vi "Autonomous Independent.vi"() -> ()   [LabVIEW 2015]
doc: "This VI is called when autonomous begins, and will automatically be terminated when autonomous ends. You can carry out timed or sensor driven robot movement independently without needing to return to the caller."
uses:
  Autonomous/Typedef/MainStates.ctl
  Autonomous/SubVI/Auton System Monitor.ctl
  Autonomous/Typedef/Defences.ctl
  Autonomous/Typedef/AutonRefType.ctl
  <vilib>/Rock Robotics/WPI/RobotDrive/WPI_RobotDriveDevRef.ctl
  <vilib>/Rock Robotics/WPI/MotorControl/WPI_MotorControlDeviceRef.ctl
  <vilib>/Rock Robotics/WPI/MotorControl/WPI_MotorControlType.ctl
  <vilib>/Rock Robotics/SystemInterfaces/DIO/FPGA_DIOPWMChannel.ctl
  <vilib>/Rock Robotics/WPI/PWM/WPI_PWMDeadband.ctl
  <vilib>/Rock Robotics/WPI/CAN/Jaguar/SubVIs/WPI_CANJaguar_ControlMode.ctl
  <vilib>/Rock Robotics/WPI/CAN/TalonSRX/WPI_CANTalonSRX_APIControlMode.ctl
  <vilib>/Rock Robotics/WPI/Encoder/WPI_EncoderDevRef.ctl
  <vilib>/Rock Robotics/SystemInterfaces/Encoder/FPGA_EncoderIdx.ctl
  <vilib>/Rock Robotics/SystemInterfaces/Counter/FPGA_CounterCtrSystemIndex.ctl
  <vilib>/Rock Robotics/WPI/Encoder/WPI_EncoderType.ctl
  <vilib>/Rock Robotics/WPI/Switch/WPI_SwitchDevRef.ctl
  <vilib>/Rock Robotics/SystemInterfaces/DIO/FPGA_DIOChannel.ctl
  NavX/TypeDefs/Z900_navX_DeviceTypeDef.ctl
  NavX/TypeDefs/Z900_navX_ProtocolTypeDef.ctl
  NavX/TypeDefs/Z900_navX_NotifyPacketTypeDef.ctl
  NavX/TypeDefs/Z900_navX_ActionTypeDef.ctl
  <vilib>/Rock Robotics/WPI/Potentiometer/WPI_PotentiometerDevRef.ctl
  <vilib>/Rock Robotics/SystemInterfaces/AI/FPGA_AIChannel.ctl
  <vilib>/Rock Robotics/Network Tables/NT Read String.vi
  <vilib>/Rock Robotics/WPI/Utilities/WPI_GetSetVariantRefNum.vi
  <vilib>/Rock Robotics/Network Tables/NT Write String.vi
  Robot Global Data.vi
  <vilib>/Rock Robotics/WPI/RobotDrive/WPI_RobotDriveArcadeDrive_Standard(NoSaturation).vi
  NavX/navX Library v2.lvlib
  <vilib>/ptbypt/NI_PtbyPt.lvlib
  ArmController/ArmController.lvlib
panel:
  in  "Channels":i32[](array[numeric]) caption="Drive Channels to Monitor"
  out "System Monitor Config":T1={"Brownout?"=FALSE, "Current Max?"=FALSE, "System Max Current"=240.0, "Min Voltage"=6.2, "Drive Motor Max Current"=40.0, "Drive Motor Time (s)"=3.5}
  out "System Monitor":T2(graph)
  in  "RUN":bool=TRUE
  in  "stop":bool
  in  "Test Case":T3
  in  "Test Case":bool
  in  "Auton Steps":T4(tab)
  in  "Gyro Turn Output Range":cluster{"output high":dbl, "output low":dbl}={"output high"=0.8, "output low"=-0.8}
  in  "Gyro PID gains":T5={"proportional gain (Kc)"=0.0005, "integral time (Ti, min)"=0.0, "derivative time (Td, min)"=0.0} {"derivative time (Td, min)" format="%.3f"; "integral time (Ti, min)" format="%.3f"; "proportional gain (Kc)" format="%.5f"}
  in  "Target Position":dbl=158.0 format="%#_13g"
  in  "Speed":dbl=0.75
  out "Encoder Difference":dbl=9.15275203438432
  out "Angle Error":dbl=0.004439899999999999
  in  "output rate (EGU/min)":dbl=1.0 format="%.2f"
  in  "Hit Wall Distance":dbl=60.0 format="%#_13g"
  in  "Hit wall speed":dbl=0.35
  in  "Gyro Turn Output Range 2":cluster{"output high":dbl, "output low":dbl}={"output high"=0.5, "output low"=-0.5}
  in  "Backup Distance":dbl=-24.0 format="%#_13g"
  in  "Hit wall speed 2":dbl=0.45
  in  "Gyro Turn Output Range 3":cluster{"output high":dbl, "output low":dbl}={"output high"=0.65, "output low"=-0.65}
  in  "Max Vel (in/s)":dbl=50.0
  in  "Kp_Yaw 2":dbl=0.0005 format="%#_13g"
  in  "Max Accel (in/s^2)":dbl=400.0
  in  "output range 3":cluster{"output high":dbl, "output low":dbl}={"output high"=0.7, "output low"=-0.7}
  in  "Kv 3":dbl=0.012
  in  "Period (s) 3":dbl=0.005
  in  "Ka 3":dbl
  in  "PID gains 3":T5
  out "Waveform Chart":T2(graph)
  in  "Kv":dbl=0.012
  in  "Ka":dbl
  in  "Period (s)":dbl=0.005
  in  "output range":cluster{"output high":dbl, "output low":dbl}={"output high"=1.0, "output low"=-1.0} {"output low" format="%.2f"; "output high" format="%.2f"}
  in  "PID gains":T5 {"derivative time (Td, min)" format="%.3f"; "integral time (Ti, min)" format="%.3f"; "proportional gain (Kc)" format="%.3f"}
  in  "Target Position 2":dbl=60.0 format="%#_13g"
  in  "Max Acceleration":dbl=400.0
  in  "Max Velocity":dbl=75.0
  in  "Kp_Yaw":dbl
  in  "Scrub Factor":dbl=0.6
  out "Waveform Chart 2":T2(graph)
  in  "Max Velocity 2":dbl=60.0
  in  "Max Acceleration 2":dbl=600.0
  in  "Target Angle (deg)":dbl=-180.0 format="%#_13g"
  in  "output range 2":cluster{"output high":dbl, "output low":dbl}={"output high"=1.0, "output low"=-1.0} {"output low" format="%.2f"; "output high" format="%.2f"}
  in  "Period (s) 2":dbl=0.005
  in  "PID gains 2":T5={"proportional gain (Kc)"=0.005, "integral time (Ti, min)"=0.0, "derivative time (Td, min)"=0.0} {"derivative time (Td, min)" format="%.3f"; "integral time (Ti, min)" format="%.3f"; "proportional gain (Kc)" format="%.3f"}
  in  "Ka 2":dbl=0.0045
  in  "Kv 2":dbl=0.012
  out "CDF":T6(graph)
  in  "CDF Pos":dbl=0.608 format="%#_13g"
  in  "Speed 1":dbl=-0.34 format="%#_13g"
  in  "CDF Detect":dbl=0.585 format="%#_13g"
  in  "Start Wait":u32=1500
  in  "Drive Time x 20ms":i32=300
  in  "Drive Val":dbl format="%#_13g"
  # "Just above motor brownout"
  # "Hit Driversation Wall"
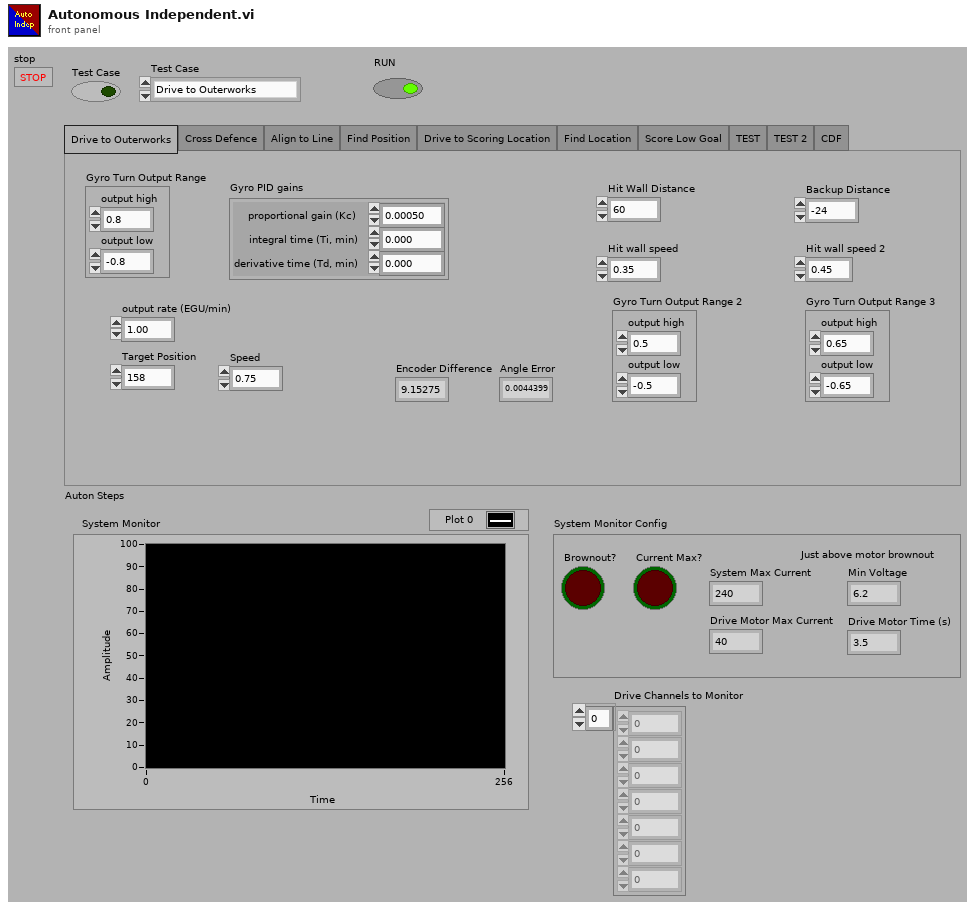
[diagram p1: front panel]
types:
  T1 = typedef "Auton System Monitor.ctl" = cluster{"Brownout?":bool, "Current Max?":bool, "System Max Current":dbl, "Min Voltage":dbl, "Drive Motor Max Current":dbl, "Drive Motor Time (s)":dbl}
  T2 = cluster{"Distance":dbl, "dx/dt":dbl, "dx/dt":dbl, "dx/dt":dbl}
  T3 = typedef "MainStates.ctl" = enum16{"Drive to Outerworks", "Cross Defence", "Align to Line", "Turn to Goal", "Find Position", "Find Distance", "Drive to Scoring Location", "Score Low Goal", "SquareToField", "Hit Driver Station Wall", "Drive Back to Position", "CDF", "Cleanup", "_TEST_Profile", "_TEST_TurnProfile", "_TEST_Impulse", "Error"}
  T4 = enum32{"Drive to Outerworks", "Cross Defence", "Align to Line", "Find Position", "Drive to Scoring Location", "Find Location", "Score Low Goal", "TEST", "TEST 2", "CDF"}
  T5 = cluster{"proportional gain (Kc)":dbl, "integral time (Ti, min)":dbl, "derivative time (Td, min)":dbl}
  T6 = cluster{"Normalized Value":dbl, "CDF Detect":dbl}
  T7 = typedef "AutonRefType.ctl" = cluster{"Starting Pos":u32, "Defence":T8, "Drivetrain":T9, "State":T3, "Encoder Right":T17, "Encoder Left":T17, "Line Sensor":T21, "navX":T23, "Front Arm":T25, "Start Time":u32, "State Vars":variant}
  T8 = typedef "Defences.ctl" = enum16{"Low Bar", "Chivel De Fris", "Sally Port", "Portcullis", "Draw Bridge", "Moat", "Rough Terrain", "Ramparts", "Rock Wall"}
  T9 = typedef "WPI_RobotDriveDevRef.ctl" = cluster{"DevStatus":errorcluster, "Motors[]":T10[], "Square Inputs":bool, "Max Output":dbl}
  T10 = typedef "WPI_MotorControlDeviceRef.ctl" = cluster{"DeviceStatus":errorcluster, "Type":T11, "PWM":cluster{"PWM Channel":T12, "DeadBand":T13}, "CAN":cluster{"Device Number":u8, "Control Mode":T14, "Semaphore":T15, "Max Vout":dbl, "TalonSRX Control Mode":T16}, "Invert":bool}
  T11 = typedef "WPI_MotorControlType.ctl" = enum16{"PWM", "CAN", "CANTalonSRX"}
  T12 = typedef "FPGA_DIOPWMChannel.ctl" = enum8{"PWM 0", "PWM 1", "PWM 2", "PWM 3", "PWM 4", "PWM 5", "PWM 6", "PWM 7", "PWM 8", "PWM 9", "PWM MXP 0", "PWM MXP 1", "PWM MXP 2", "PWM MXP 3", "PWM MXP 4", "PWM MXP 5", "PWM MXP 6", "PWM MXP 7", "PWM MXP 8", "PWM MXP 9", "Invalid"}
  T13 = typedef "WPI_PWMDeadband.ctl" = cluster{"Name":string, "maxPositivePwm":i32, "minPositivePwm":i32, "centerPwm":i32, "maxNegativePwm":i32, "minNegativePwm":i32, "angularRange":u16}
  T14 = typedef "WPI_CANJaguar_ControlMode.ctl" = enum8{"Percent VBus", "Current", "Speed", "Position", "Voltage"}
  T15 = typedef "Semaphore RefNum" = refnum<k1>
  T16 = typedef "WPI_CANTalonSRX_APIControlMode.ctl" = enum8{"Percent VBus", "Speed", "Position", "Slave", "Unchanged / Invalid", "Voltage Compensation", "Current", "Motion Profile"}
  T17 = typedef "WPI_EncoderDevRef.ctl" = cluster{"DevStatus":errorcluster, "EncoderIndex":T18, "CounterIndex":T19, "DistancePerCount":dbl, "Decoding Type":T20}
  T18 = typedef "FPGA_EncoderIdx.ctl" = enum8{"Enc 0", "Enc 1", "Enc 2", "Enc 3", "Enc 4", "Enc 5", "Enc 6", "Enc 7", "Invalid"}
  T19 = typedef "FPGA_CounterCtrSystemIndex.ctl" = enum8{"Ctr 0", "Ctr 1", "Ctr 2", "Ctr 3", "Ctr 4", "Ctr 5", "Ctr 6", "Ctr 7", "Invalid"}
  T20 = typedef "WPI_EncoderType.ctl" = enum16{"1x", "2x", "4x"}
  T21 = typedef "WPI_SwitchDevRef.ctl" = cluster{"DevStatus":errorcluster, "DIO Channel":T22, "CntIndex":T19, "Normally Closed":bool}
  T22 = typedef "FPGA_DIOChannel.ctl" = enum8{"DIO 0", "DIO 1", "DIO 2", "DIO 3", "DIO 4", "DIO 5", "DIO 6", "DIO 7", "DIO 8", "DIO 9", "DIO MXP 0", "DIO MXP 1", "DIO MXP 2", "DIO MXP 3", "DIO MXP 4", "DIO MXP 5", "DIO MXP 6", "DIO MXP 7", "DIO MXP 8", "DIO MXP 9", "DIO MXP 10", "DIO MXP 11", "DIO MXP 12", "DIO MXP 13", "DIO MXP 14", "DIO MXP 15", "Invalid"}
  T23 = typedef "navX Library v2.lvlib/Z900_navX_DeviceTypeDef.ctl" = cluster{"Interface":cluster{"Protocol":T24, "Update Rate (4Hz-60Hz)":u8, "navX Open TypeDef":variant}, "Notify Packet":refnum<notifier>, "Loop VI Refnum":refnum<vi>, "Ready to Close Occurrence Refnum":refnum<k4>}
  T24 = typedef "navX Library v2.lvlib/Z900_navX_ProtocolTypeDef.ctl" = enum16{"SERIAL", "I2C", "SPI"}
  T25 = typedef "WPI_PotentiometerDevRef.ctl" = cluster{"DevStatus":errorcluster, "Analog Channel":T26, "Invert Output":bool}
  T26 = typedef "FPGA_AIChannel.ctl" = enum8{"AI 0", "AI 1", "AI 2", "AI 3", "AI MXP 0", "AI MXP 1", "AI MXP 2", "AI MXP 3", "Invalid"}
  T27 = typedef "Motion Profile.ctl" = cluster{"Position":dbl[], "Velocity":dbl[], "Time":dbl[], "Acceleration":dbl[]}
  T28 = cluster{"Yaw":dbl, "Roll":dbl, "Pitch":dbl, "Heading":dbl, "Fused Heading":dbl}
  T29 = cluster{"Down":dbl, "Pickup":dbl, "Shoot":dbl, "Turtle":dbl, "Intake Transfer":dbl, "Hang":dbl}
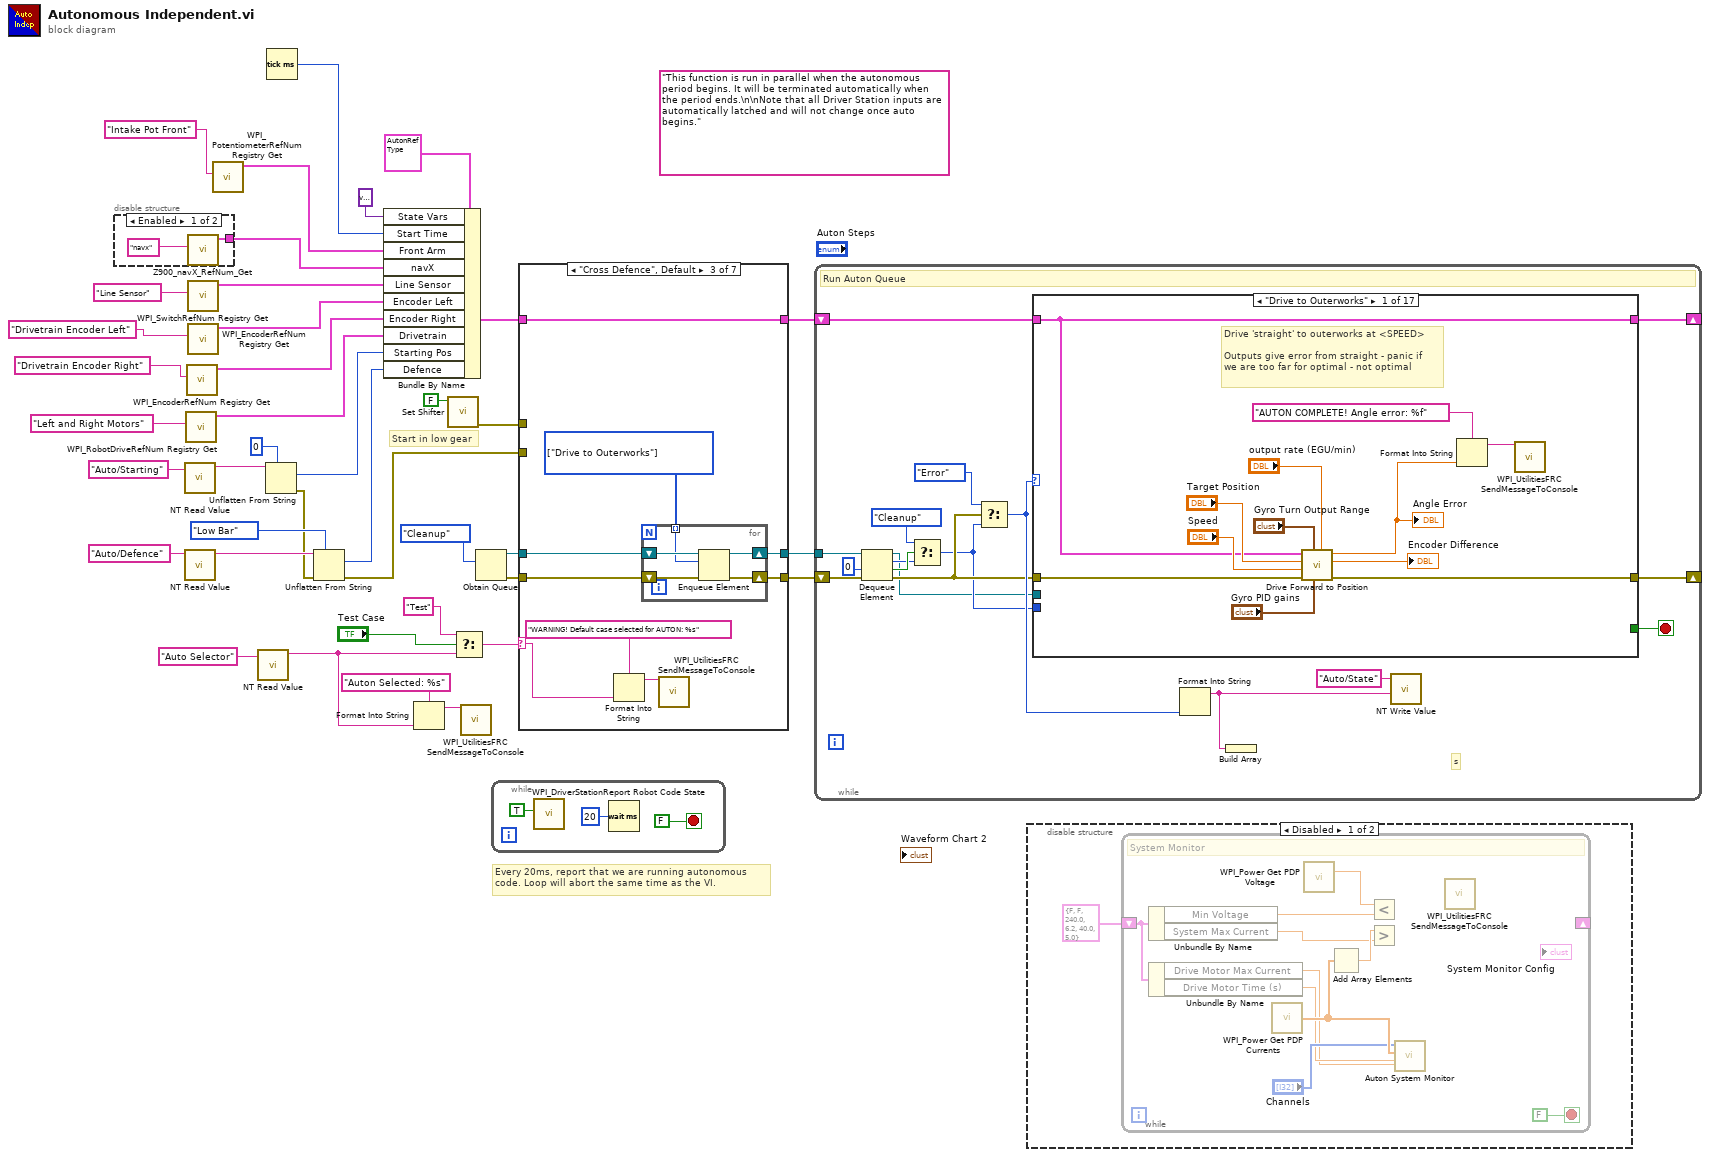
[diagram p0: block diagram]
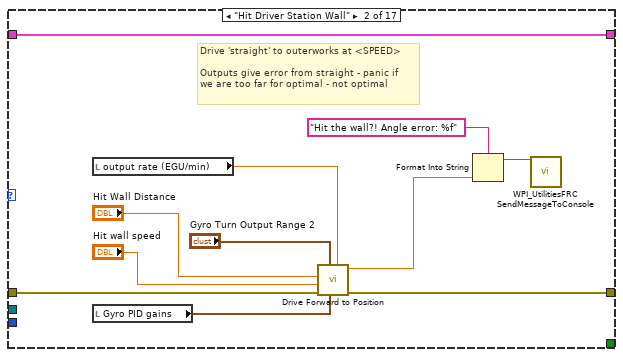
[diagram p4: hidden frame]
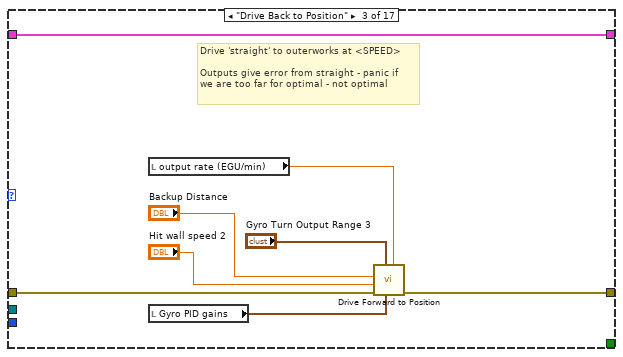
[diagram p5: hidden frame]
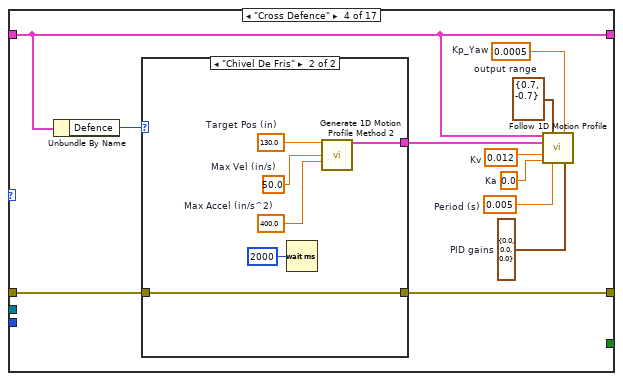
[diagram p6: hidden frame]
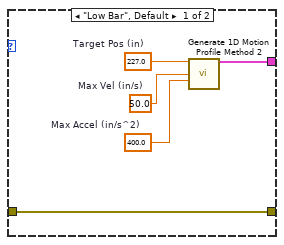
[diagram p7: hidden frame]
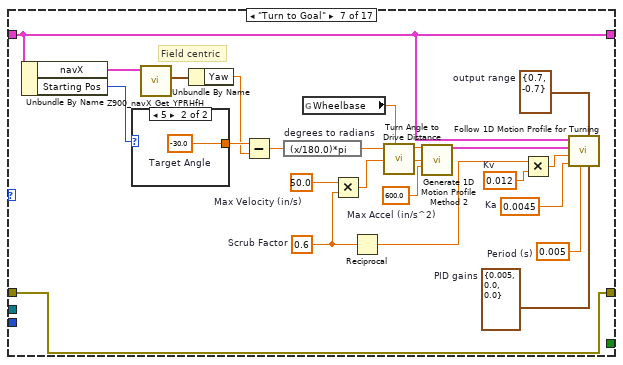
[diagram p10: hidden frame]
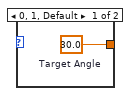
[diagram p11: hidden frame]
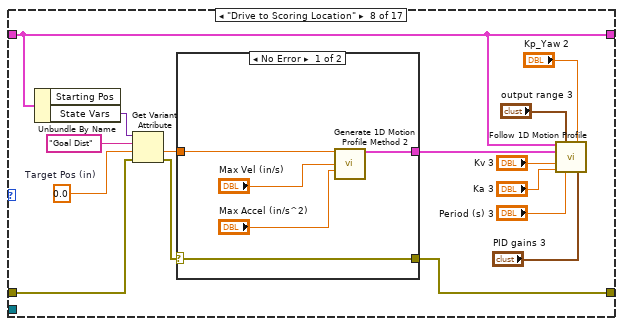
[diagram p12: hidden frame]
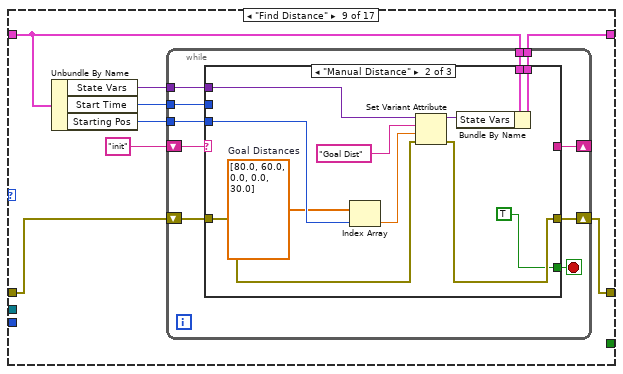
[diagram p14: hidden frame]
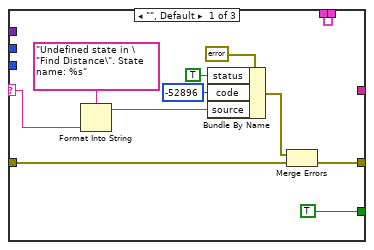
[diagram p15: hidden frame]
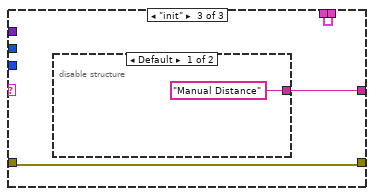
[diagram p16: hidden frame]
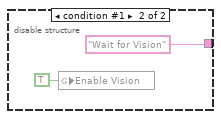
[diagram p17: hidden frame]
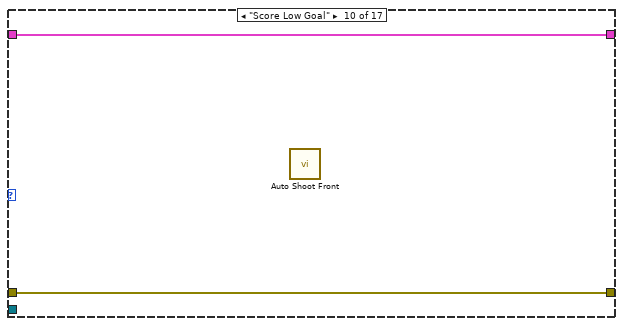
[diagram p18: hidden frame]
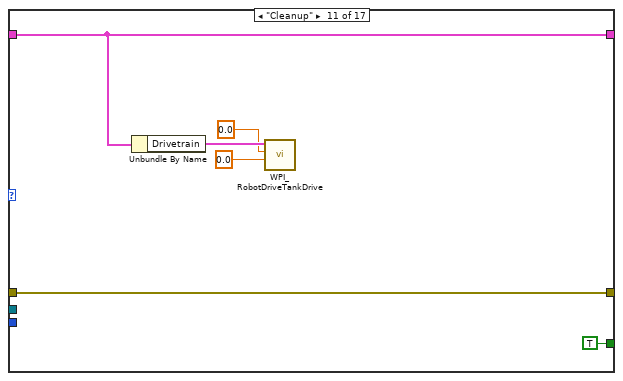
[diagram p19: hidden frame]
diagram:
  (unwired) "This function is run in parallel when the autonomous period begins. It will be terminated automatically when the period ends.\n\nNote that all Driver Station inputs are automatically latched and will not change once auto begins."
  # "Start in low gear"
  # "Every 20ms, report that we are running autonomous\ncode. Loop will abort the same time as the VI."
  n1 = disable-structure shown="Enabled" {
    disable-tunnel: [w41 _] -> w23
    frame Enabled {
      n2 = call "Z900_navX_RefNum_Get.vi"("refnum name"="navx") -> ("navX Device"=w41:T23)  [unwired: 9 in, 1 out]
    }
    frame Disabled {
    }
  }
  n3 = call-poly <vilib>:"NT Read Value.vi"("Name"="Auto/Starting") -> ("String"=w36:string)  [unwired: 9 in, 1 out]
  n4 = call-poly <vilib>:"NT Read Value.vi"("Name"="Auto/Defence") -> ("String"=w37:string)  [unwired: 9 in, 1 out]
  n5 = call <vilib>:"WPI_RobotDriveRefNum Registry Get.vi"("refnum name"="Left and Right Motors") -> ("RobotDriveDevRef"=w29:T9)  [unwired: 1 in, 9 out]
  n6 = call <vilib>:"WPI_EncoderRefNum Registry Get.vi"("refnum name"="Drivetrain Encoder Right") -> ("EncoderDevRef"=w26:T17)  [unwired: 9 in, 1 out]
  n7 = call <vilib>:"WPI_SwitchRefNum Registry Get.vi"("refnum name"="Line Sensor") -> ("SwitchDevRef"=w25:T21)  [unwired: 9 in, 1 out]
  n8 = call <vilib>:"WPI_EncoderRefNum Registry Get.vi"("refnum name"="Drivetrain Encoder Left") -> ("EncoderDevRef"=w27:T17)  [unwired: 9 in, 1 out]
  n9 = call <vilib>:"WPI_PotentiometerRefNum Registry Get.vi"("refnum name"="Intake Pot Front") -> ("PotDevRef"=w3:T25)  [unwired: 9 in, 1 out]
  n10 = call-poly <vilib>:"NT Read Value.vi"("Name"="Auto Selector") -> ("String"=w7:string)  [unwired: 9 in, 1 out]
  n11 = Unflatten From String(type=u32 0, binary string=w36) -> (value=w31:u32, error out=w20:errorcluster)  [unwired: 3 in, 1 out]
  n12 = Tick Count (ms)() -> (millisecond timer value=w2:u32)
  n13 = Unflatten From String(type=Defences."Low Bar", binary string=w37, error in (no error)=w20) -> (value=w32:T8, error out=w13:errorcluster)  [unwired: 2 in, 1 out]
  n14 = Bundle By Name(cluster=T7 {"Starting Pos"=0, "Defence"=enum."Chivel De Fris", "Drivetrain"={"DevStatus"={"status"=FALSE, "code"=0, "source"=""}, "Motors[]"=[], "Square Inputs"=FALSE, "Max Output"=1.0}, "State"=enum."Drive to Outerworks", "Encoder Right"={"DevStatus"={"status"=FALSE, "code"=0, "source"=""}, "EncoderIndex"=enum."Invalid", "CounterIndex"=enum."Invalid", "DistancePerCount"=1.0, "Decoding Type"=enum."4x"}, "Encoder Left"={"DevStatus"={"status"=FALSE, "code"=0, "source"=""}, "EncoderIndex"=enum."Invalid", "CounterIndex"=enum."Invalid", "DistancePerCount"=1.0, "Decoding Type"=enum."4x"}, "Line Sensor"={"DevStatus"={"status"=FALSE, "code"=0, "source"=""}, "DIO Channel"=enum."Invalid", "CntIndex"=enum."Invalid", "Normally Closed"=FALSE}, "navX"={"Interface"={"Protocol"=enum."SERIAL", "Update Rate (4Hz-60Hz)"=4, "navX Open TypeDef"=variant}, "Notify Packet"=refnum, "Loop VI Refnum"=refnum, "Ready to Close Occurrence Refnum"=refnum}, "Front Arm"={"DevStatus"={"status"=FALSE, "code"=0, "source"=""}, "Analog Channel"=enum."Invalid", "Invert Output"=FALSE}, "Start Time"=0, "State Vars"=variant}, "State Vars"=variant, "Start Time"=w2, "Front Arm"=w3, "navX"=w23, "Line Sensor"=w25, "Encoder Left"=w27, "Encoder Right"=w26, "Drivetrain"=w29, "Starting Pos"=w31, "Defence"=w32) -> (w28:T7)
  n15 = Format Into String(format string="Auton Selected: %s", w7) -> (resulting string=w5:string)  [unwired: 2 in, 1 out]
  n16 = call "Set Shifter.vi"("Gear (F = Low Gear)"=FALSE) -> ("error out"=w10:errorcluster)  [unwired: 10 in]
  n17 = Select(t="Test", s="Test Case", f=w7) -> (s? t:f=w8:string)
  n18 = call <vilib>:"WPI_UtilitiesFRC SendMessageToConsole.vi"("Message"=w5) -> ()  [unwired: 14 in, 1 out]
  n19 = Obtain Queue(element data type=MainStates."Cleanup" ("State")) -> (queue out=w15:refnum<queue>, error out=w16:errorcluster)  [unwired: 4 in, 1 out]
  n20 = while {
    stop <- FALSE stop-if-true
    n21 = call <vilib>:"WPI_DriverStationReport Robot Code State.vi"("Autonomous"=TRUE) -> ()  [unwired: 10 in, 1 out]
    n22 = Wait (ms)(milliseconds to wait=u32 20) -> ()  [unwired: 1 out]
  }
  n23 = case shown="\"Cross Defence\", Default" w8 {
    selector: w8 -> [_ _ w67 w81 _ _ _]
    tunnel: w28 -> [w51 w63 w75 w89 w100 w111 w125]
    tunnel: [w51 w63 w75 w89 w100 w111 w119] -> w22
    tunnel: [w49 w60 w71 w85 w96 w107 w121] -> w21
    tunnel: w16 -> [w48 w64 w73 w87 w98 w109 w123]
    tunnel: [w47 w62 w72 w86 w97 w108 w122] -> w19
    tunnel: w15 -> [w46 w61 w74 w88 w99 w110 w124]
    tunnel: w13 -> [_ _ _ _ _ _ _]
    tunnel: w10 -> [_ _ _ _ _ _ _]
    frame "Score Low Goal" {
      # "Queue Actions for Auton Routine"
      n24 = disable-structure shown="Disabled" {
        disable-tunnel: [w52 _] -> w50
        frame Disabled {
          w52 = T3[] [enum."Drive to Outerworks", enum."Cross Defence", enum."Align to Line", enum."Find Position", enum."Drive to Scoring Location", enum."Find Distance", enum."Score Low Goal", enum."Cleanup"] items=["Drive to Outerworks", "Cross Defence", "Align to Line", "Turn to Goal", "Find Position", "Find Distance", "Drive to Scoring Location", "Score Low Goal", "SquareToField", "Hit Driver Station Wall", "Drive Back to Position", "CDF", "Cleanup", "_TEST_Profile", "_TEST_TurnProfile", "_TEST_Impulse", "Error"]
        }
        frame Enabled {
        }
      }
      n25 = for {
        tunnel: w50 -> [w56] mode=indexing
        shift-right: [w55] -> w49
        shift-left: w46 -> [w57]
        shift-right: [w53] -> w47
        shift-left: w48 -> [w54]
        n26 = Enqueue Element(queue=w57, element=w56, error in (no error)=w54) -> (queue out=w55:refnum<queue>, error out=w53:errorcluster)  [unwired: 1 in, 1 out]
      }
    }
    frame "Test" {
      n27 = while {
        stop <- "RUN" stop-if-true
        n28 = Wait (ms)(milliseconds to wait=u32 100) -> ()  [unwired: 1 out]
      }
      n29 = Enqueue Element(queue=w61, element="Test Case", error in (no error)=w64) -> (queue out=w60:refnum<queue>, error out=w62:errorcluster)  [unwired: 1 in, 1 out]
      n30 = call <vilib>:"WPI_UtilitiesFRC SendMessageToConsole.vi"("Message"="WARNING! Test case selected for AUTON" ("format string")) -> ()  [unwired: 14 in, 1 out]
    }
    frame "Cross Defence", Default {
      w70 = T3[] [enum."Drive to Outerworks"] items=["Drive to Outerworks", "Cross Defence", "Align to Line", "Turn to Goal", "Find Position", "Find Distance", "Drive to Scoring Location", "Score Low Goal", "SquareToField", "Hit Driver Station Wall", "Drive Back to Position", "CDF", "Cleanup", "_TEST_Profile", "_TEST_TurnProfile", "_TEST_Impulse", "Error"]
      n31 = Format Into String(format string="WARNING! Default case selected for AUTON: %s", w67) -> (resulting string=w69:string)  [unwired: 2 in, 1 out]
      n32 = for {
        tunnel: w70 -> [w79] mode=indexing
        shift-right: [w78] -> w71
        shift-left: w74 -> [w80]
        shift-right: [w76] -> w72
        shift-left: w73 -> [w77]
        n33 = Enqueue Element(queue=w80, element=w79, error in (no error)=w77) -> (queue out=w78:refnum<queue>, error out=w76:errorcluster)  [unwired: 1 in, 1 out]
      }
      n34 = call <vilib>:"WPI_UtilitiesFRC SendMessageToConsole.vi"("Message"=w69) -> ()  [unwired: 14 in, 1 out]
    }
    frame "CFLG" {
      w84 = T3[] [enum."Drive to Outerworks", enum."Hit Driver Station Wall", enum."Drive Back to Position", enum."Turn to Goal", enum."Find Distance", enum."Drive to Scoring Location", enum."Score Low Goal"] items=["Drive to Outerworks", "Cross Defence", "Align to Line", "Turn to Goal", "Find Position", "Find Distance", "Drive to Scoring Location", "Score Low Goal", "SquareToField", "Hit Driver Station Wall", "Drive Back to Position", "CDF", "Cleanup", "_TEST_Profile", "_TEST_TurnProfile", "_TEST_Impulse", "Error"]
      n35 = Format Into String(format string="WARNING! Default case selected for AUTON: %s", w81) -> (resulting string=w83:string)  [unwired: 2 in, 1 out]
      n36 = for {
        tunnel: w84 -> [w93] mode=indexing
        shift-right: [w92] -> w85
        shift-left: w88 -> [w94]
        shift-right: [w90] -> w86
        shift-left: w87 -> [w91]
        n37 = Enqueue Element(queue=w94, element=w93, error in (no error)=w91) -> (queue out=w92:refnum<queue>, error out=w90:errorcluster)  [unwired: 1 in, 1 out]
      }
      n38 = call <vilib>:"WPI_UtilitiesFRC SendMessageToConsole.vi"("Message"=w83) -> ()  [unwired: 14 in, 1 out]
    }
    frame "CDF Auto" {
      w95 = T3[] [enum."CDF", enum."Cleanup"] items=["Drive to Outerworks", "Cross Defence", "Align to Line", "Turn to Goal", "Find Position", "Find Distance", "Drive to Scoring Location", "Score Low Goal", "SquareToField", "Hit Driver Station Wall", "Drive Back to Position", "CDF", "Cleanup", "_TEST_Profile", "_TEST_TurnProfile", "_TEST_Impulse", "Error"]
      n39 = for {
        tunnel: w95 -> [w104] mode=indexing
        shift-right: [w103] -> w96
        shift-left: w99 -> [w105]
        shift-right: [w101] -> w97
        shift-left: w98 -> [w102]
        n40 = Enqueue Element(queue=w105, element=w104, error in (no error)=w102) -> (queue out=w103:refnum<queue>, error out=w101:errorcluster)  [unwired: 1 in, 1 out]
      }
    }
    frame "Do Nothing" {
      w106 = T3[] [enum."Cleanup"] items=["Drive to Outerworks", "Cross Defence", "Align to Line", "Turn to Goal", "Find Position", "Find Distance", "Drive to Scoring Location", "Score Low Goal", "SquareToField", "Hit Driver Station Wall", "Drive Back to Position", "CDF", "Cleanup", "_TEST_Profile", "_TEST_TurnProfile", "_TEST_Impulse", "Error"]
      n41 = for {
        tunnel: w106 -> [w115] mode=indexing
        shift-right: [w114] -> w107
        shift-left: w110 -> [w116]
        shift-right: [w112] -> w108
        shift-left: w109 -> [w113]
        n42 = Enqueue Element(queue=w116, element=w115, error in (no error)=w113) -> (queue out=w114:refnum<queue>, error out=w112:errorcluster)  [unwired: 1 in, 1 out]
      }
    }
    frame "Low Bar Score" {
      # "No Camera Low Goal from Low Bar"
      n43 = disable-structure shown="Enabled" {
        disable-tunnel: [w126 w127 w128 _] -> w120
        frame Enabled {
          w126 = T3[] [enum."Cross Defence", enum."Turn to Goal"] items=["Drive to Outerworks", "Cross Defence", "Align to Line", "Turn to Goal", "Find Position", "Find Distance", "Drive to Scoring Location", "Score Low Goal", "SquareToField", "Hit Driver Station Wall", "Drive Back to Position", "CDF", "Cleanup", "_TEST_Profile", "_TEST_TurnProfile", "_TEST_Impulse", "Error"]
        }
        frame Disabled {
          w127 = T3[] [enum."Cross Defence", enum."Turn to Goal"] items=["Drive to Outerworks", "Cross Defence", "Align to Line", "Turn to Goal", "Find Position", "Find Distance", "Drive to Scoring Location", "Score Low Goal", "SquareToField", "Hit Driver Station Wall", "Drive Back to Position", "CDF", "Cleanup", "_TEST_Profile", "_TEST_TurnProfile", "_TEST_Impulse", "Error"]
        }
        frame Disabled {
          w128 = T3[] [enum."Cross Defence", enum."Turn to Goal", enum."Drive to Scoring Location", enum."Score Low Goal"] items=["Drive to Outerworks", "Cross Defence", "Align to Line", "Turn to Goal", "Find Position", "Find Distance", "Drive to Scoring Location", "Score Low Goal", "SquareToField", "Hit Driver Station Wall", "Drive Back to Position", "CDF", "Cleanup", "_TEST_Profile", "_TEST_TurnProfile", "_TEST_Impulse", "Error"]
        }
        frame Disabled {
        }
      }
      n44 = for {
        tunnel: w120 -> [w132] mode=indexing
        shift-right: [w131] -> w121
        shift-left: w124 -> [w133]
        shift-right: [w129] -> w122
        shift-left: w123 -> [w130]
        n45 = Enqueue Element(queue=w133, element=w132, error in (no error)=w130) -> (queue out=w131:refnum<queue>, error out=w129:errorcluster)  [unwired: 1 in, 1 out]
      }
      n46 = Bundle By Name(cluster=w125, "Defence"=Defences."Low Bar", "Starting Pos"=u32 0) -> (w119:T7)
    }
  }
  n47 = while {
    shift-right: [w149] -> _
    shift-left: w22 -> [w135]
    tunnel: w21 -> [w146]
    shift-right: [w137] -> _
    shift-left: w19 -> [w145]
    stop <- w150 stop-if-true
    # "s"
    # "Run Auton Queue"
    n48 = Dequeue Element(queue=w146, timeout in ms (-1)=0, error in (no error)=w145) -> (queue out=w136:refnum<queue>, element=w140:T3, timed out?=w141:bool, error out=w143:errorcluster)
    n49 = Select(t=MainStates."Cleanup", s=w141, f=w140) -> (s? t:f=w138:T3)
    n50 = Select(t=MainStates."Error", s=w143, f=w138) -> (s? t:f=w144:T3)
    n51 = case shown="\"Drive to Outerworks\"" w144 {
      tunnel: w135 -> [w151 w163 w174 w184 w205 w207 w214 w241 w255 w301 w305 w309 w311 w404 w415 w433 w448]
      tunnel: [_ _ _ _ _ _ _ _ _ _ TRUE _ _ _ _ _ _] -> w150
      tunnel: [w151 w163 w174 w184 w205 w207 w214 w241 w254 w301 w305 w309 w311 w404 w415 w433 w448] -> w149
      tunnel: w143 -> [w162 w173 w181 w192 w204 w206 w215 w234 w259 w300 w306 w308 w312 w403 w422 w440 w449]
      tunnel: w138 -> [_ _ _ _ _ _ _ _ _ _ _ _ _ w392 _ _ _]
      tunnel: [w161 w172 w180 w190 w204 w206 w215 w233 w258 w300 w306 w308 w312 w390 w422 w440 w449] -> w137
      tunnel: w136 -> [_ _ _ _ _ _ _ _ _ _ _ _ _ w391 _ _ _]
      frame "Drive to Outerworks" {
        # "Drive 'straight' to outerworks at <SPEED>\n\nOutputs give error from straight - panic if\nwe are too far for optimal - not optimal"
        n52 = call "Drive Forward to Position.vi"("output rate (EGU/min)"="output rate (EGU/min)", "PID gains"="Gyro PID gains", "output range"="Gyro Turn Output Range", "error in (no error)"=w162, "Speed"="Speed", "Target"="Target Position", "AutonRef"=w151) -> ("error out"=w161:errorcluster, "Encoder Difference"=→"Encoder Difference":dbl, "Angle Error"=w153:dbl)  [unwired: 2 in]
        "Angle Error" <- w153
        n53 = Format Into String(format string="AUTON COMPLETE! Angle error: %f", w153) -> (resulting string=w154:string)  [unwired: 2 in, 1 out]
        n54 = call <vilib>:"WPI_UtilitiesFRC SendMessageToConsole.vi"("Message"=w154) -> ()  [unwired: 14 in, 1 out]
      }
      frame "Hit Driver Station Wall" {
        # "Drive 'straight' to outerworks at <SPEED>\n\nOutputs give error from straight - panic if\nwe are too far for optimal - not optimal"
        n55 = local read "output rate (EGU/min)"() -> (w164:dbl)
        n56 = local read "Gyro PID gains"() -> (w165:T5)
        n57 = call "Drive Forward to Position.vi"("output rate (EGU/min)"=w164, "PID gains"=w165, "output range"="Gyro Turn Output Range 2", "error in (no error)"=w173, "Speed"="Hit wall speed", "Target"="Hit Wall Distance") -> ("error out"=w172:errorcluster, "Angle Error"=w167:dbl)  [unwired: 3 in, 1 out]
        n58 = Format Into String(format string="Hit the wall?! Angle error: %f", w167) -> (resulting string=w168:string)  [unwired: 2 in, 1 out]
        n59 = call <vilib>:"WPI_UtilitiesFRC SendMessageToConsole.vi"("Message"=w168) -> ()  [unwired: 14 in, 1 out]
      }
      frame "Drive Back to Position" {
        # "Drive 'straight' to outerworks at <SPEED>\n\nOutputs give error from straight - panic if\nwe are too far for optimal - not optimal"
        n60 = local read "output rate (EGU/min)"() -> (w175:dbl)
        n61 = local read "Gyro PID gains"() -> (w176:T5)
        n62 = call "Drive Forward to Position.vi"("output rate (EGU/min)"=w175, "PID gains"=w176, "output range"="Gyro Turn Output Range 3", "error in (no error)"=w181, "Speed"="Hit wall speed 2", "Target"="Backup Distance") -> ("error out"=w180:errorcluster)  [unwired: 3 in, 2 out]
      }
      frame "Cross Defence" {
        w182 = 0.0005  # Kp_Yaw
        w188 = cluster{"output high":dbl, "output low":dbl} {"output high"=0.7, "output low"=-0.7}  # output range
        w186 = T5 {"proportional gain (Kc)"=0.0, "integral time (Ti, min)"=0.0, "derivative time (Td, min)"=0.0}  # PID gains
        w187 = 0.005  # Period (s)
        w189 = 0.0  # Ka
        w185 = 0.012  # Kv
        n63 = Unbundle By Name(w184) -> ("Defence"=w191:T8)
        n64 = case shown="\"Chivel De Fris\"" w191 {
          tunnel: w192 -> [w197 w203]
          tunnel: [w197 w203] -> w190
          tunnel: [w193 w199] -> w183
          frame "Low Bar", Default {
            w196 = 50.0  # Max Vel (in/s)
            w195 = 400.0  # Max Accel (in/s^2)
            w194 = 227.0  # Target Pos (in)
            n65 = call "Generate 1D Motion Profile Method 2.vi"("Target Position"=w194, "Max Velocity"=w196, "Max Acceleration"=w195) -> ("Profile Plot"=w193:T27)  [unwired: 11 in, 1 out]
          }
          frame "Chivel De Fris" {
            w202 = 50.0  # Max Vel (in/s)
            w201 = 400.0  # Max Accel (in/s^2)
            w200 = 130.0  # Target Pos (in)
            n66 = Wait (ms)(milliseconds to wait=u32 2000) -> ()  [unwired: 1 out]
            n67 = call "Generate 1D Motion Profile Method 2.vi"("Target Position"=w200, "Max Velocity"=w202, "Max Acceleration"=w201) -> ("Profile Plot"=w199:T27)  [unwired: 11 in, 1 out]
          }
        }
        n68 = call "Follow 1D Motion Profile.vi"("auton ref"=w184, "output range"=w188, "Kp_Yaw"=w182, "Profile"=w183, "Kv"=w185, "Ka"=w189, "Period (s)"=w187, "PID gains"=w186) -> ()  [unwired: 8 in]
      }
      frame "Align to Line" {
      }
      frame "Find Position" {
      }
      frame "Turn to Goal" {
        w220 = cluster{"output high":dbl, "output low":dbl} {"output high"=0.7, "output low"=-0.7}  # output range
        w221 = 0.0045  # Ka
        w219 = 0.005  # Period (s)
        w218 = T5 {"proportional gain (Kc)"=0.005, "integral time (Ti, min)"=0.0, "derivative time (Td, min)"=0.0}  # PID gains
        w217 = 0.012  # Kv
        w228 = 0.6  # Scrub Factor
        w222 = 600.0  # Max Accel (in/s^2)
        w223 = 50.0  # Max Velocity (in/s)
        # "Field centric"
        n69 = Unbundle By Name(w214) -> ("navX"=w213:T23, "Starting Pos"=w208:u32)
        n70 = case shown="5" w208 {
          tunnel: [w231 w232] -> w210
          frame 0, 1, Default {
            w231 = 30.0  # Target Angle
          }
          frame 5 {
            w232 = -30.0  # Target Angle
          }
        }
        n71 = call "Z900_navX_Get_YPRHfH.vi"("navX Device"=w213) -> ("YRPHfH"=w212:T28)  [unwired: 7 in, 3 out]
        n72 = Unbundle By Name(w212) -> ("Yaw"=w209:dbl)
        n73 = Subtract(x=w210, y=w209) -> (x-y=w211:dbl)
        n74 = expression code="(x/180.0)*pi" "degrees to radians"(w211) -> (w226:dbl)
        n75 = global read "Robot Global Data.vi" "Wheelbase"() -> (w224:dbl)
        n76 = Multiply(x=w223, y=w228) -> (x*y=w227:dbl)
        n77 = Reciprocal(x=w228) -> (1/x=w230:dbl)
        n78 = call "Turn Angle to Drive Distance.vi"("Wheelbase (in)"=w224, "Angle (rads)"=w226) -> ("Distance (in)"=w225:dbl)  [unwired: 7 in]
        n79 = call "Generate 1D Motion Profile Method 2.vi"("Target Position"=w225, "Max Velocity"=w227, "Max Acceleration"=w222) -> ("Profile Plot"=w216:T27)  [unwired: 11 in, 1 out]
        n80 = Multiply(x=w230, y=w217) -> (x*y=w229:dbl)
        n81 = call "Follow 1D Motion Profile for Turning.vi"("PID gains"=w218, "Period (s)"=w219, "output range"=w220, "Ka"=w221, "Kv"=w229, "Profile"=w216, "auton ref"=w214) -> ()  [unwired: 5 in]
      }
      frame "Drive to Scoring Location" {
        w237 = 0.0  # Target Pos (in)
        n82 = Unbundle By Name(w241) -> ("State Vars"=w239:variant)  [unwired: 1 out]
        n83 = Get Variant Attribute(Variant=w239, name="Goal Dist", default value (empty Variant)=w237, error in=w234) -> (value=w236:dbl, error out=w235:errorcluster)  [unwired: 2 out]
        n84 = case shown="No Error" w235 {
          selector: w235 -> [w248 w253]
          tunnel: [w250 _] -> w240
          tunnel: w236 -> [w249 _]
          tunnel: [w248 w253] -> w233
          frame No Error {
            n85 = call "Generate 1D Motion Profile Method 2.vi"("Target Position"=w249, "Max Velocity"="Max Vel (in/s)", "Max Acceleration"="Max Accel (in/s^2)") -> ("Profile Plot"=w250:T27)  [unwired: 11 in, 1 out]
          }
          frame Error {
          }
        }
        n86 = call "Follow 1D Motion Profile.vi"("auton ref"=w241, "output range"="output range 3", "Kp_Yaw"="Kp_Yaw 2", "Profile"=w240, "Kv"="Kv 3", "Ka"="Ka 3", "Period (s)"="Period (s) 3", "PID gains"="PID gains 3") -> ()  [unwired: 8 in]
      }
      frame "Find Distance" {
        n87 = Unbundle By Name(w255) -> ("State Vars"=w256:variant, "Start Time"=w260:u32, "Starting Pos"=w257:u32)
        n88 = while {
          shift-right: [w270] -> _
          shift-left: "init" -> [w271]
          tunnel: w260 -> [w269]
          shift-right: [w267] -> w258
          shift-left: w259 -> [w268]
          tunnel: w257 -> [w265]
          tunnel: w256 -> [w264]
          tunnel: w255 -> [w263]
          tunnel: [w262] -> w254
          stop <- w266 stop-if-true
          n89 = case shown="\"Manual Distance\"" w271 {
            selector: w271 -> [w276 _ _]
            tunnel: [_ _ w296] -> w270
            tunnel: w269 -> [_ _ _]
            tunnel: w268 -> [w280 w285 w295]
            tunnel: [w279 w284 w295] -> w267
            tunnel: [TRUE TRUE _] -> w266
            tunnel: w265 -> [_ w293 _]
            tunnel: w264 -> [_ w288 _]
            tunnel: w263 -> [w272 w291 w294]
            tunnel: [w272 w290 w294] -> w262
            frame "", Default {
              n90 = Format Into String(format string="Undefined state in \"Find Distance\". State name: %s" ("source"), w276) -> (resulting string=w275:string)  [unwired: 2 in, 1 out]
              n91 = Bundle By Name(cluster=errorcluster {"status"=FALSE, "code"=0, "source"=""} ("error constant"), "status"=TRUE, "code"=-52896, "source"=w275) -> (w278:errorcluster)
              n92 = Merge Errors(w278, w280) -> (w279:errorcluster)
            }
            frame "Manual Distance" {
              w292 = dbl[] [80.0, 60.0, 0.0, 0.0, 30.0]  # Goal Distances
              n93 = Index Array(array=w292, index=w293) -> (element=w287:dbl)
              n94 = Set Variant Attribute(Variant=w288, name="Goal Dist", value=w287, error in=w285) -> (Variant out=w289:variant, error out=w284:errorcluster)  [unwired: 1 out]
              n95 = Bundle By Name(cluster=w291, "State Vars"=w289) -> (w290:T7)
            }
            frame "init" {
              n96 = disable-structure shown="Default" {
                disable-tunnel: ["Manual Distance" "Wait for Vision"] -> w296
                frame condition #0 (active) {
                }
                frame condition #1 {
                  n97 = global write "Robot Global Data.vi" "Enable Vision"(TRUE ("Enable Vision")) -> ()
                }
              }
            }
          }
        }
      }
      frame "Score Low Goal" {
        n98 = call "Auto Shoot Front.vi"() -> ()  [unwired: 12 in]
      }
      frame "Cleanup" {
        n99 = Unbundle By Name(w305) -> ("Drivetrain"=w304:T9)
        n100 = call <vilib>:"WPI_RobotDriveTankDrive.vi"("Right axis value"=0.0, "Left axis value"=0.0, "RobotDriveDevRef"=w304) -> ()  [unwired: 6 in, 3 out]
      }
      frame "SquareToField" {
      }
      frame "CDF" {
        n101 = while {
          tunnel: w311 -> [w315]
          shift-right: [w314] -> _
          shift-left: "start" -> [w316]
          stop <- w313 stop-if-true
          n102 = case shown="\"arm down\"" w316 {
            tunnel: w315 -> [w321 w328 w335 w341 w350 w356 _ _ w378]
            tunnel: [_ "drive back slightly" "arm down" "cross CDF arm up" "stop" _ "stop" "drive to CDF" w380] -> w314
            tunnel: [TRUE _ _ _ _ _ _ _ _] -> w313
            frame "stop", Default {
              n103 = Unbundle By Name(w321) -> ("Drivetrain"=w320:T9)
              n104 = call <vilib>:"WPI_RobotDriveMotors.vi"("RightSpeed"=0.0, "LeftSpeed"=0.0, "RobotDriveDevRef"=w320) -> ()  [unwired: 6 in, 3 out]
              n105 = Wait (ms)(milliseconds to wait=u32 1500) -> ()  [unwired: 1 out]
            }
            frame "stop and wait" {
              n106 = Unbundle By Name(w328) -> ("Drivetrain"=w327:T9)
              n107 = call <vilib>:"WPI_RobotDriveMotors.vi"("RightSpeed"=0.0, "LeftSpeed"=0.0, "RobotDriveDevRef"=w327) -> ()  [unwired: 6 in, 3 out]
              n108 = Wait (ms)(milliseconds to wait=u32 500) -> ()  [unwired: 1 out]
            }
            frame "drive back slightly" {
              n109 = Unbundle By Name(w335) -> ("Drivetrain"=w334:T9)
              n110 = call <vilib>:"WPI_RobotDriveMotors.vi"("RightSpeed"=0.2, "LeftSpeed"=0.2, "RobotDriveDevRef"=w334) -> ("RobotDriveDevRef"=w330:T9)  [unwired: 6 in, 2 out]
              n111 = call <vilib>:"WPI_RobotDriveDelayAndUpdateSafety.vi"("Delay (s)"=0.5, "RobotDriveDevRef"=w330) -> ()  [unwired: 8 in, 2 out]
            }
            frame "cross CDF" {
              w336 = -0.3 ("LeftSpeed")
              n112 = Unbundle By Name(w341) -> ("Drivetrain"=w340:T9)
              n113 = call <vilib>:"WPI_RobotDriveMotors.vi"("RightSpeed"=w336, "LeftSpeed"=w336, "RobotDriveDevRef"=w340) -> ("RobotDriveDevRef"=w338:T9)  [unwired: 6 in, 2 out]
              n114 = call <vilib>:"WPI_RobotDriveDelayAndUpdateSafety.vi"("Delay (s)"=1.5, "RobotDriveDevRef"=w338) -> ()  [unwired: 8 in, 2 out]
            }
            frame "cross CDF arm up" {
              w345 = -0.3 ("LeftSpeed")
              n115 = Unbundle By Name(w350) -> ("Drivetrain"=w349:T9)
              n116 = call "Front Arm Positions.vi"() -> ("Front Arm"=w343:T29)  [unwired: 10 in, 1 out]
              n117 = Unbundle By Name(w343) -> ("Turtle"=w342:dbl)
              n118 = call "Set Arm.vi"("Intake"=enum16{"Front", "Rear"}."Front", "Position"=w342) -> ()  [unwired: 10 in]
              n119 = call <vilib>:"WPI_RobotDriveMotors.vi"("RightSpeed"=w345, "LeftSpeed"=w345, "RobotDriveDevRef"=w349) -> ("RobotDriveDevRef"=w347:T9)  [unwired: 6 in, 2 out]
              n120 = call <vilib>:"WPI_RobotDriveDelayAndUpdateSafety.vi"("Delay (s)"=2.5, "RobotDriveDevRef"=w347) -> ()  [unwired: 8 in, 2 out]
            }
            frame "arm down" {
              n121 = call "Front Arm Positions.vi"() -> ("Front Arm"=w358:T29)  [unwired: 10 in, 1 out]
              n122 = Unbundle By Name(w356) -> ("Front Arm"=w355:T25)
              n123 = Unbundle By Name(w358) -> ("Down"=w357:dbl)
              n124 = call "Set Arm.vi"("Intake"=enum16{"Front", "Rear"}."Front", "Position"=w357) -> ()  [unwired: 10 in]
              n125 = flat-sequence {
                tunnel: w355 -> [w360]
                tunnel: [w360] -> w354
                tunnel: w354 -> [w365]
                tunnel: [w362] -> w353
                frame #0 {
                  n126 = Wait (ms)(milliseconds to wait=u32 1000) -> ()  [unwired: 1 out]
                }
                frame #1 {
                  n127 = call <vilib>:"WPI_PotentiometerGetNormalized.vi"("PotDevRef"=w365) -> ("Normalized Value"=w364:dbl)  [unwired: 8 in, 2 out]
                  n128 = Greater?(x=w364, y="Drive Val") -> (0:w362:bool)
                }
              }
              n129 = Select(t="cross CDF", s=w353, f="arm up stop") -> ()  [unwired: 1 out]
            }
            frame "arm up stop" {
              n130 = call "Front Arm Positions.vi"() -> ("Front Arm"=w368:T29)  [unwired: 10 in, 1 out]
              n131 = Unbundle By Name(w368) -> ("Turtle"=w367:dbl)
              n132 = call "Set Arm.vi"("Intake"=enum16{"Front", "Rear"}."Front", "Position"=w367) -> ()  [unwired: 10 in]
            }
            frame "start" {
              n133 = call "Set Arm.vi"("Intake"=enum16{"Front", "Rear"}."Front", "Position"="CDF Pos") -> ()  [unwired: 10 in]
              n134 = Wait (ms)(milliseconds to wait="Start Wait") -> ()  [unwired: 1 out]
            }
            frame "drive to CDF" {
              n135 = Unbundle By Name(w378) -> ("Drivetrain"=w375:T9)
              n136 = Unbundle By Name(w378) -> ("Front Arm"=w377:T25)
              n137 = for {
                N: "Drive Time x 20ms" -> [_]
                tunnel: w377 -> [w389]
                tunnel: [w388] -> w376
                tunnel: w375 -> [w386]
                stop <- w388 stop-if-true
                n138 = call <vilib>:"WPI_PotentiometerGetNormalized.vi"("PotDevRef"=w389) -> ("Normalized Value"=w384:dbl)  [unwired: 8 in, 2 out]
                n139 = call <vilib>:"WPI_RobotDriveMotors.vi"("RightSpeed"="Speed 1", "LeftSpeed"="Speed 1", "RobotDriveDevRef"=w386) -> ()  [unwired: 6 in, 3 out]
                n140 = Less?(x=w384, y="CDF Detect") -> (x < y?=w388:bool)
                n141 = Wait (ms)(milliseconds to wait=u32 20) -> ()  [unwired: 1 out]
                n142 = Bundle("Normalized Value"=w384, "CDF Detect"="CDF Detect") -> (→"CDF":T6)  [unwired: 1 in]
              }
              n143 = Select(t="stop and drop", s=w376, f="stop") -> (s? t:f=w380:string)
            }
          }
        }
      }
      frame "Error" {
        # "Filter errors here"
        n144 = Unbundle By Name(w403) -> ("status"=w402:bool, "code"=w398:i32, "source"=w397:string)
        n145 = Select(t="ERROR!", s=w402, f="Warning!") -> (s? t:f=w399:string)
        n146 = Format Into String(format string="%s Recieved in AUTON. Code: %d %s", w399, w398, w397) -> (resulting string=w395:string)  [unwired: 2 in, 1 out]
        n147 = call <vilib>:"WPI_UtilitiesFRC SendMessageToConsole.vi"("Message"=w395, "error in (no error)"=w403) -> ("error out"=w394:errorcluster)  [unwired: 13 in]
        n148 = Unbundle By Name(w394) -> ("code"=w393:i32)
        n149 = case shown="0" w393 {
          tunnel: w392 -> [w405 _]
          tunnel: w391 -> [w406 w409]
          tunnel: [w407 w410] -> w390
          frame 0 {
            # "Queue prev state"
            n150 = Enqueue Element(queue=w406, element=w405) -> (error out=w407:errorcluster)  [unwired: 2 in, 2 out]
          }
          frame Default {
            # "Default to cleanup"
            n151 = Enqueue Element(queue=w409, element=MainStates."Cleanup") -> (error out=w410:errorcluster)  [unwired: 2 in, 2 out]
          }
        }
      }
      frame "_TEST_Profile" {
        n152 = call "Generate 1D Motion Profile Method 2.vi"("Target Position"="Target Position 2", "Max Velocity"="Max Velocity", "Max Acceleration"="Max Acceleration") -> ("Profile Plot"=w412:T27)  [unwired: 11 in, 1 out]
        n153 = call "Follow 1D Motion Profile.vi"("auton ref"=w415, "output range"="output range", "Kp_Yaw"="Kp_Yaw", "Profile"=w412, "Kv"="Kv", "Ka"="Ka", "Period (s)"="Period (s)", "PID gains"="PID gains") -> ()  [unwired: 8 in]
      }
      frame "_TEST_TurnProfile" {
        n154 = global read "Robot Global Data.vi" "Wheelbase"() -> (w430:dbl)
        n155 = expression code="(x/180.0)*pi" "degrees to radians"("Target Angle (deg)") -> (w427:dbl)
        n156 = Multiply(x="Scrub Factor", y="Max Velocity 2") -> (x*y=w426:dbl)
        n157 = Reciprocal(x="Scrub Factor") -> (1/x=w423:dbl)
        n158 = call "Turn Angle to Drive Distance.vi"("Wheelbase (in)"=w430, "Angle (rads)"=w427) -> ("Distance (in)"=w428:dbl)  [unwired: 7 in]
        n159 = call "Generate 1D Motion Profile Method 2.vi"("Target Position"=w428, "Max Velocity"=w426, "Max Acceleration"="Max Acceleration 2") -> ("Profile Plot"=w439:T27)  [unwired: 11 in, 1 out]
        n160 = Multiply(x=w423, y="Kv 2") -> (x*y=w424:dbl)
        n161 = call "Follow 1D Motion Profile for Turning.vi"("PID gains"="PID gains 2", "Period (s)"="Period (s) 2", "output range"="output range 2", "Ka"="Ka 2", "Kv"=w424, "Profile"=w439, "auton ref"=w433) -> ()  [unwired: 5 in]
      }
      frame "_TEST_Impulse" {
        n162 = Unbundle By Name(w448) -> ("Drivetrain"=w441:T9, "Encoder Right"=w444:T17)
        n163 = while {
          tunnel: w444 -> [w460]
          tunnel: w441 -> [w452]
          stop <- "stop" stop-if-true
          w454 = 0.005 ("dt")
          n164 = call <vilib>:"WPI_EncoderGet.vi"("EncoderDevRef"=w460) -> ("Distance"=w458:dbl)  [unwired: 5 in, 5 out]
          n165 = Unbundle By Name(w452) -> ("Motors[]"=w451:T10[])
          n166 = Index Array(array=w451) -> (element=w450:T10)  [unwired: 1 in]
          n167 = call <vilib>:"Derivative x(t) PtByPt.vi"("dt"=w454, "x"=w458) -> ("dx/dt"=w457:dbl)  [unwired: 2 in, 1 out]
          n168 = call <vilib>:"Derivative x(t) PtByPt.vi"("dt"=w454, "x"=w457) -> ("dx/dt"=w456:dbl)  [unwired: 2 in, 1 out]
          n169 = call <vilib>:"WPI_MotorControlGetOutput.vi"("MotorControlDevRef"=w450) -> ()  [unwired: 8 in, 3 out]
          n170 = call <vilib>:"Derivative x(t) PtByPt.vi"("dt"=w454, "x"=w456) -> ("dx/dt"=w455:dbl)  [unwired: 2 in, 1 out]
          n171 = Bundle("Distance"=w458, "dx/dt"=w457, "dx/dt"=w456, "dx/dt"=w455) -> (→"Waveform Chart":T2)  [unwired: 1 in]
          n172 = Wait (ms)(milliseconds to wait=u32 5) -> ()  [unwired: 1 out]
        }
        n173 = call-poly <vilib>:"WPI_RobotDriveArcadeDrive.vi"("Y axis value"=-1.0, "RobotDriveDevRef"=w441) -> ("RobotDriveDevRef"=w446:T9)  [unwired: 7 in, 2 out]
        n174 = call <vilib>:"WPI_RobotDriveDelayAndUpdateSafety.vi"("Delay (s)"=1.0, "RobotDriveDevRef"=w446) -> ("RobotDriveDevRef 2"=w443:T9)  [unwired: 8 in, 1 out]
        n175 = call-poly <vilib>:"WPI_RobotDriveArcadeDrive.vi"("Y axis value"=0.0, "RobotDriveDevRef"=w443) -> ()  [unwired: 7 in, 3 out]
      }
    }
    n176 = Format Into String(w144) -> (resulting string=w134:string)  [unwired: 3 in, 1 out]
    n177 = Build Array(w134) -> ()  [unwired: 1 out]
    n178 = call-poly <vilib>:"NT Write Value.vi"("String"=w134, "Name"="Auto/State") -> ()  [unwired: 9 in, 1 out]
  }
  n179 = disable-structure shown="Disabled" {
    frame Disabled {
      n180 = while {
        shift-right: _ -> [_]
        shift-left: T1 {"Brownout?"=FALSE, "Current Max?"=FALSE, "System Max Current"=240.0, "Min Voltage"=6.2, "Drive Motor Max Current"=40.0, "Drive Motor Time (s)"=5.0} ("System Monitor Config") -> [w467]
        stop <- FALSE stop-if-true
        # "System Monitor"
        n181 = Unbundle By Name(w467) -> ("Min Voltage"=w470:dbl, "System Max Current"=w468:dbl)
        n182 = Unbundle By Name(w467) -> ("Drive Motor Max Current"=w463:dbl, "Drive Motor Time (s)"=w464:dbl)
        n183 = call <vilib>:"WPI_Power Get PDP Currents.vi"() -> ("all currents (A)"=w466:dbl[])  [unwired: 13 in, 2 out]
        n184 = call <vilib>:"WPI_Power Get PDP Voltage.vi"() -> ("voltage (V)"=w471:dbl)  [unwired: 14 in, 1 out]
        n185 = Add Array Elements(numeric array=w466) -> (sum=w469:dbl)
        n186 = Less?(x=w471, y=w470) -> ()  [unwired: 1 out]
        n187 = Greater?(x=w469, y=w468) -> ()  [unwired: 1 out]
        n188 = call "Auton System Monitor.vi"(6:w463, 9:w464, "all currents (A)"=w466, "Channels"="Channels") -> ()  [unwired: 8 in]
        n189 = call <vilib>:"WPI_UtilitiesFRC SendMessageToConsole.vi"() -> ()  [unwired: 15 in, 1 out]
      }
    }
    frame Enabled {
    }
  }
